vi "Discover Tests.vi"(8 "error in (no error)":errorcluster, 11 "Unit Tests for Runner in":refnum<class "Unit Tests for Runner.lvclass">) -> (0 "error out":errorcluster, 3 "Unit Tests for Runner out":refnum<class "Unit Tests for Runner.lvclass">)   [LabVIEW 2013, in "Unit Tests for Runner.lvclass"]
uses:
  Unit Tests for Runner.lvclass
  classes/Test Runner/Test Runner.lvclass
  support files/root define test.vi
  support files/lone test.vi
  classes/Test/Test.lvclass
  classes/Assert/Assert.lvclass
panel:
  out "Pass?":bool
  out "Test VIs":path[](array[path])
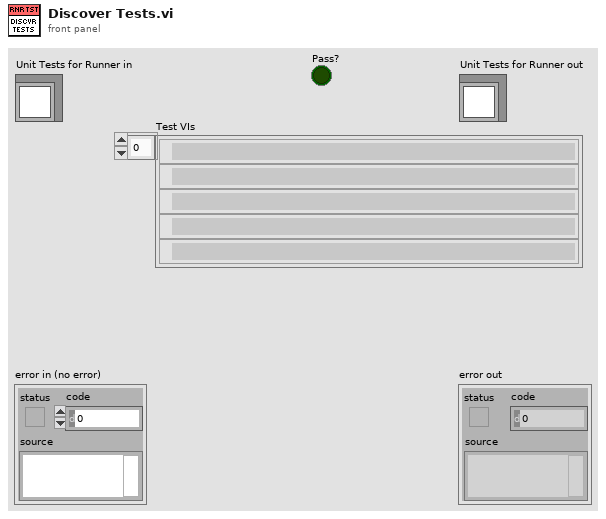
[diagram p1: front panel]
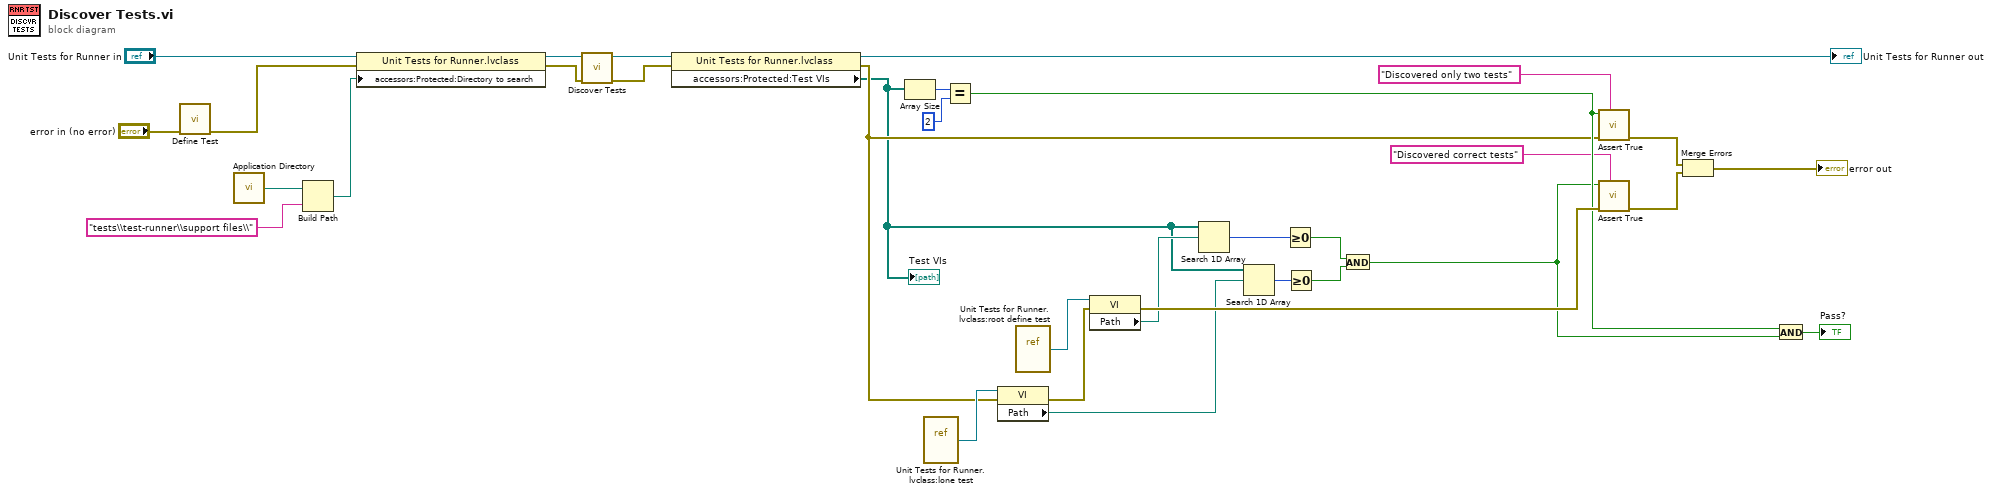
[diagram p0: block diagram]
diagram:
  n1 = call "Define Test.vi"("error in (no error)"="error in (no error)") -> ("error out"=w20:errorcluster)  [unwired: 10 in]
  n2 = call <vilib>:"Application Directory.vi"() -> ("Application Directory"=w31:path)
  n3 = Build Path(base path=w31, name or relative path="tests\\test-runner\\support files\\") -> (appended path=w28:path)
  n4 = property class="Unit Tests for Runner.lvclass"(reference="Unit Tests for Runner in", error in=w20, "accessors:Protected:Directory to search"=w28) -> (reference out=w29:refnum<class "Unit Tests for Runner.lvclass">, error out=w27:errorcluster)
  n5 = call-parent "Discover Tests.vi"("error in (no error)"=w27, "Test Runner in"=w29) -> ("error out"=w26:errorcluster, "Test Runner out"=w25:refnum<class "Unit Tests for Runner.lvclass">)  [unwired: 8 in]
  n6 = property class="Unit Tests for Runner.lvclass"(reference=w25, error in=w26) -> (reference out=→"Unit Tests for Runner out":refnum<class "Unit Tests for Runner.lvclass">, error out=w10:errorcluster, "accessors:Protected:Test VIs"=w7:path[])
  "Test VIs" <- w7
  n7 = Array Size(array=w7) -> (size(s)=w23:i32)
  n8 = vi-ref "Unit Tests for Runner.lvclass:lone test.vi"() -> (w11:refnum<vi>)
  n9 = Equal?(x=w23, y=2) -> (x = y?=w15:bool)
  n10 = property class="VI"(reference=w11, error in=w10) -> (error out=w9:errorcluster, "Path"=w6:path)  [unwired: 1 out]
  n11 = vi-ref "Unit Tests for Runner.lvclass:root define test.vi"() -> (w21:refnum<vi>)
  n12 = property class="VI"(reference=w21, error in=w9) -> (error out=w19:errorcluster, "Path"=w8:path)  [unwired: 1 out]
  n13 = Search 1D Array(1D array=w7, element=w8) -> (index of element=w5:i32)  [unwired: 1 in]
  n14 = Search 1D Array(1D array=w7, element=w6) -> (index of element=w4:i32)  [unwired: 1 in]
  n15 = Greater Or Equal To 0?(x=w5) -> (x >= 0?=w3:bool)
  n16 = Greater Or Equal To 0?(x=w4) -> (x >= 0?=w2:bool)
  n17 = And(x=w3, y=w2) -> (x .and. y?=w1:bool)
  n18 = call "Assert True.vi"("Label"="Discovered only two tests", "error in (no error)"=w10, "True?"=w15) -> ("error out"=w18:errorcluster)  [unwired: 8 in]
  n19 = call "Assert True.vi"("Label"="Discovered correct tests", "error in (no error)"=w19, "True?"=w1) -> ("error out"=w17:errorcluster)  [unwired: 8 in]
  n20 = Merge Errors(w18, w17) -> (→"error out":errorcluster)
  n21 = And(x=w15, y=w1) -> (x .and. y?=→"Pass?":bool)
